vi "2DGaussianfun.vi"(3 "output control":T1, 4 "data":variant, 5 "X":dbl[](array[numeric]), 6 "Coefficients":dbl[](array[numeric])) -> (0 "error out":errorcluster, 1 "f'(X,a)":dbl[][](array[numeric]), 2 "f(X,a)":dbl[](array[numeric]))   [LabVIEW 2014]
uses:
  <vilib>/gmath/NumericalOptimization/LM_output select.ctl
  <vilib>/gmath/NI_Gmath.lvlib
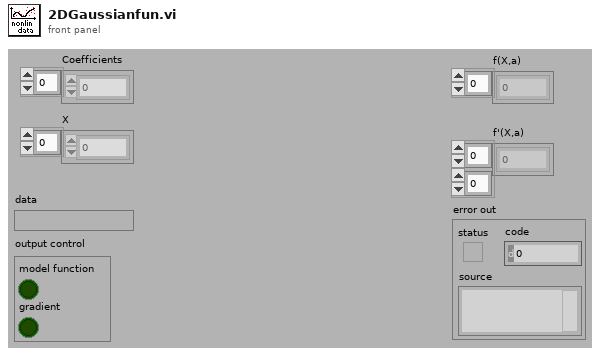
[diagram p1: front panel]
types:
  T1 = typedef "NI_Gmath.lvlib/LM_output select.ctl" = cluster{"model function":bool, "gradient":bool}
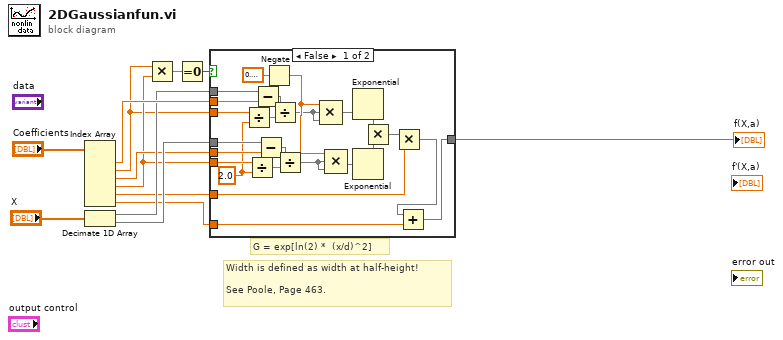
[diagram p0: block diagram]
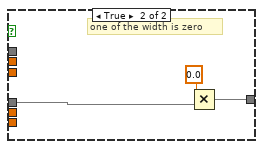
[diagram p2: hidden frame]
diagram:
  # "G = exp[ln(2) *  (x/d)^2]"
  # "Width is defined as width at half-height!\n\nSee Poole, Page 463."
  n1 = Index Array(array="Coefficients") -> (element #1=w13:dbl, element #2=w5:dbl, element #3=w10:dbl, element #4=w9:dbl, element #5=w4:dbl, element #6=w1:dbl)  [unwired: 6 in]
  n2 = Decimate 1D Array("X") -> (w12:dbl[], w11:dbl[])
  n3 = Multiply(x=w5, y=w9) -> (x*y=w8:dbl)
  n4 = Equal To 0?(x=w8) -> (x = 0?=w7:bool)
  n5 = case shown="False" w7 {
    tunnel: w13 -> [w37 _]
    tunnel: w12 -> [w36 _]
    tunnel: w5 -> [w35 _]
    tunnel: w11 -> [w34 w38]
    tunnel: w10 -> [w33 _]
    tunnel: w9 -> [w30 _]
    tunnel: [w14 w39] -> w2
    tunnel: w4 -> [w27 _]
    tunnel: w1 -> [w15 _]
    frame False {
      w28 = 2.0 ("y")
      n6 = Divide(x=w35, y=w28) -> (x/y=w31:dbl)
      n7 = Divide(x=w30, y=w28) -> (x/y=w29:dbl)
      n8 = Subtract(x=w36, y=w37) -> (x-y=w22:dbl[])
      n9 = Subtract(x=w34, y=w33) -> (x-y=w21:dbl[])
      n10 = Negate(x=0.6931471805599453) -> (-x=w25:dbl)
      n11 = Divide(x=w22, y=w31) -> (x/y=w23:dbl[])
      n12 = Divide(x=w21, y=w29) -> (x/y=w20:dbl[])
      n13 = Compound Arithmetic op=MULTIPLY(w25, w23, w23) -> (w24:dbl[])
      n14 = Compound Arithmetic op=MULTIPLY(w25, w20, w20) -> (w19:dbl[])
      n15 = Exponential(1:w24) -> (0:w17:dbl[])
      n16 = Exponential(1:w19) -> (0:w18:dbl[])
      n17 = Multiply(x=w17, y=w18) -> (x*y=w32:dbl[])
      n18 = Multiply(x=w32, y=w27) -> (x*y=w16:dbl[])
      n19 = Add(x=w16, y=w15) -> (x+y=w14:dbl[])
    }
    frame True {
      # "one of the width is zero"
      n20 = Multiply(x=0.0, y=w38) -> (x*y=w39:dbl[])
    }
  }
  "f(X,a)" <- w2
